vi "Keithley 2220A 2230A 2231A Set Voltage and Current Limit.vi"(0 "VISA resource name":refnum<visa-resource-name>, 1 "ID Query? (T: Yes)":bool, 2 "Reset? (T: Yes)":bool, 5 "Channel Control":u16(ring)=1 items=["N/A", "Channel 1", "Channel 2", "Channel 3"], 7 "Supply Voltage":dbl=5.0, 9 "Output Current":dbl=1.0, 11 "error in (no error)":errorcluster, 12 "Output State":u16(ring) items=["OFF", "ON"]) -> (4 "VISA resource name out":refnum<visa-resource-name>, 6 "Instr ID":string, 8 "Measured Voltage":sgl, 10 "Measured Current":sgl, 15 "error out":errorcluster)   [LabVIEW 2019]
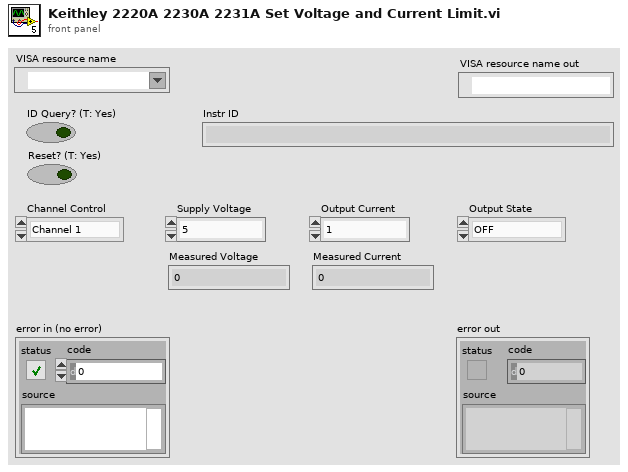
[diagram p1: front panel]
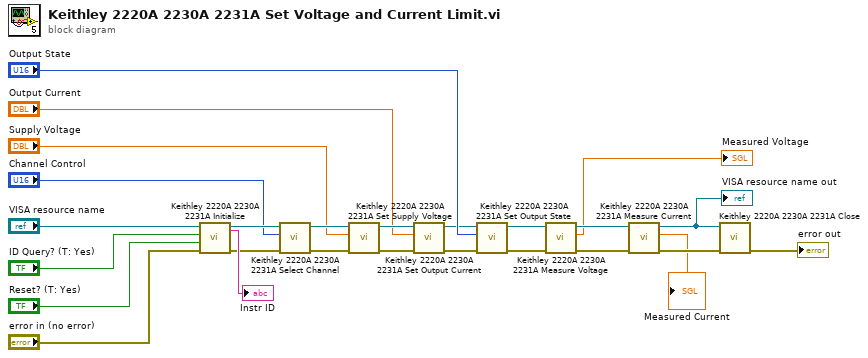
[diagram p0: block diagram]
diagram:
  n1 = call "Keithley 2220A 2230A 2231A Initialize.vi"("error in (no error)"="error in (no error)", "Reset? (T: Yes)"="Reset? (T: Yes)", "ID Query? (T: Yes)"="ID Query? (T: Yes)", "VISA resource name"="VISA resource name") -> ("error out"=w20:errorcluster, "VISA resource name out"=w19:refnum<visa-resource-name>, "Instr ID"=→"Instr ID":string)  [unwired: 5 in]
  n2 = call "Keithley 2220A 2230A 2231A Select Channel.vi"("error in (no error)"=w20, "Channel Control"="Channel Control", "VISA resource name"=w19) -> ("error out"=w15:errorcluster, "VISA resource name out"=w16:refnum<visa-resource-name>)  [unwired: 7 in]
  n3 = call "Keithley 2220A 2230A 2231A Set Supply Voltage.vi"("error in (no error)"=w15, "Supply Voltage"="Supply Voltage", "VISA resource name"=w16) -> ("error out"=w12:errorcluster, "VISA resource name out"=w13:refnum<visa-resource-name>)  [unwired: 7 in]
  n4 = call "Keithley 2220A 2230A 2231A Set Output Current.vi"("error in (no error)"=w12, "Output Current"="Output Current", "VISA resource name"=w13) -> ("error out"=w9:errorcluster, "VISA resource name out"=w10:refnum<visa-resource-name>)  [unwired: 7 in]
  n5 = call "Keithley 2220A 2230A 2231A Set Output State.vi"("error in (no error)"=w9, "Channel Control"="Output State", "VISA resource name"=w10) -> ("error out"=w5:errorcluster, "VISA resource name out"=w8:refnum<visa-resource-name>)  [unwired: 7 in]
  n6 = call "Keithley 2220A 2230A 2231A Measure Voltage.vi"("error in (no error)"=w5, "VISA resource name"=w8) -> ("error out"=w6:errorcluster, "Measured Voltage"=→"Measured Voltage":sgl, "VISA resource name out"=w7:refnum<visa-resource-name>)  [unwired: 7 in]
  n7 = call "Keithley 2220A 2230A 2231A Measure Current.vi"("error in (no error)"=w6, "VISA resource name"=w7) -> ("error out"=w3:errorcluster, "Measured Current"=→"Measured Current":sgl, "VISA resource name out"=w4:refnum<visa-resource-name>)  [unwired: 7 in]
  "VISA resource name out" <- w4
  n8 = call "Keithley 2220A 2230A 2231A Close.vi"("error in (no error)"=w3, "VISA resource name"=w4) -> ("error out"=→"error out":errorcluster)  [unwired: 9 in]
